vi "Write To SQL.vi"(1 "SQL query":string, 2 "connection information":string) -> (0 "error out":errorcluster)   [LabVIEW 2014]
uses:
  <vilib>/addons/database/Connection.llb/DB Tools Open Connec (String).vi
  <vilib>/addons/database/Connection.llb/Conn Execute.vi
  <vilib>/addons/database/Recordset.llb/Rec Destroy - Connection.vi
  <vilib>/addons/database/NI_Database_API.lvlib
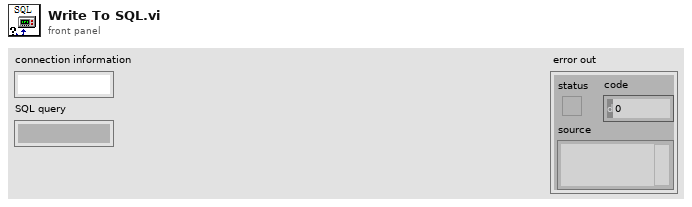
[diagram p1: front panel]
types:
  T1 = typedef "NI_Database_API.lvlib/Conn ObjectReference.ctl" = refnum<k1>
  T2 = typedef "NI_Database_API.lvlib/Rec ObjectReference.ctl" = refnum<k1>
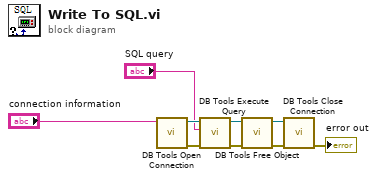
[diagram p0: block diagram]
diagram:
  n1 = call-poly <vilib>:"DB Tools Open Connection.vi"("connection information"="connection information") -> ("error out"=w7:errorcluster, "connection reference"=w8:T1)  [unwired: 7 in]
  n2 = call-poly <vilib>:"DB Tools Execute Query.vi"("error in (no error)"=w7, "SQL query"="SQL query", "connection reference"=w8) -> ("error out"=w4:errorcluster, "recordset reference"=w5:T2)  [unwired: 5 in]
  n3 = call-poly <vilib>:"DB Tools Free Object.vi"("error in (no error)"=w4, "recordset reference"=w5) -> ("error out"=w2:errorcluster, "connection reference"=w3:T1)  [unwired: 8 in]
  n4 = call <vilib>:"DB Tools Close Connection.vi"("error in (no error)"=w2, "connection reference"=w3) -> ("error out"=→"error out":errorcluster)  [unwired: 5 in]
